vi "Calc_Force_Moment_Balance_ver2.vi"(8 "Center State at T":T2, 9 "Ini_Anchor_Posi":dbl[][](array[numeric]), 10 "Torque":dbl, 11 "On_Particle State":T1(array[cluster])) -> (0 "New Center State at T":T2, 1 "Ini_Anchor_Posi":dbl[][](array[numeric]), 2 "Rot_angle":dbl, 3 "On_Particle State":T1(array[cluster]), 4 "final Moment":dbl, 6 "initial Moment":dbl)   [LabVIEW 2020]
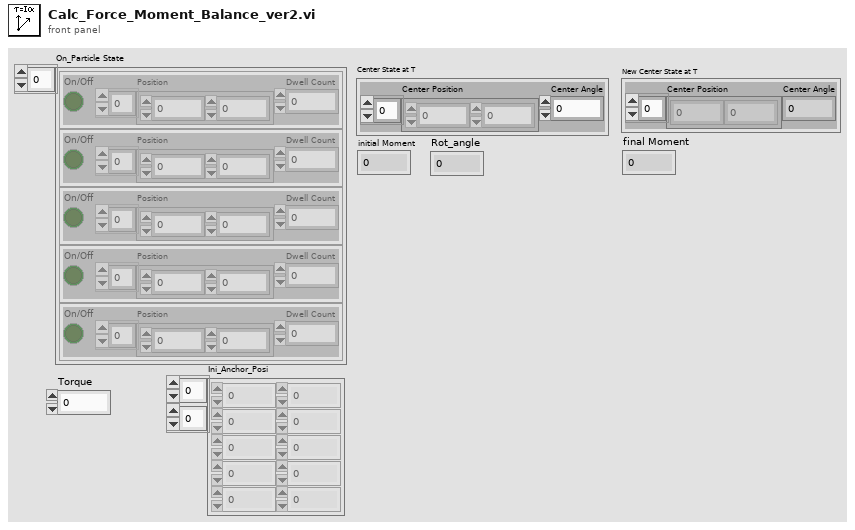
[diagram p1: front panel]
types:
  T1 = cluster{"On/Off":bool, "Position":dbl[], "Dwell Count":i32}[]
  T2 = cluster{"Center Position":dbl[], "Center Angle":dbl}
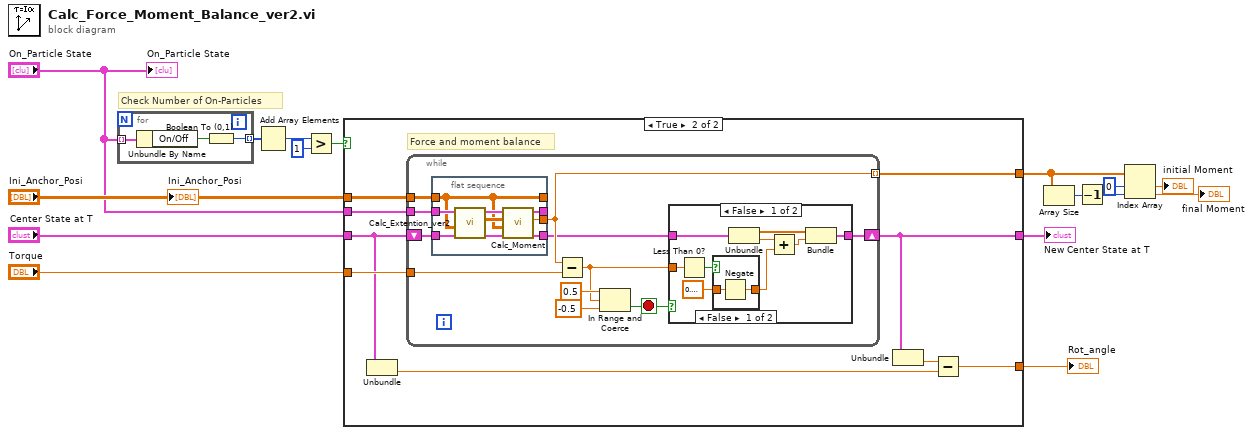
[diagram p0: block diagram]
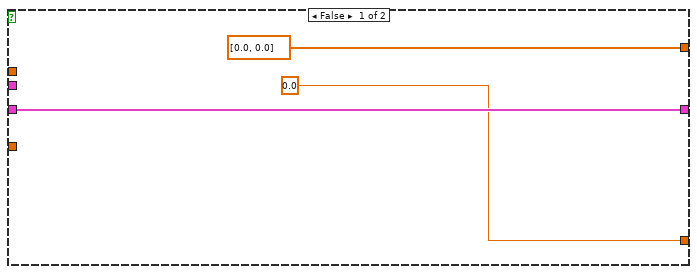
[diagram p2: hidden frame]
diagram:
  # "Check Number of On-Particles"
  n1 = for {
    tunnel: "On_Particle State" -> [w19] mode=indexing
    tunnel: [w17] -> w15 mode=indexing
    n2 = Unbundle By Name(w19) -> ("On/Off"=w18:bool)
    n3 = Boolean To (0,1)(Boolean=w18) -> (0, 1=w17:i16)
  }
  n4 = Add Array Elements(numeric array=w15) -> (sum=w9:i16)
  n5 = Greater?(x=w9, y=i16 1) -> (0:w13:bool)
  n6 = case shown="TRUE" w13 {
    tunnel: "Center State at T" -> [w22 w25]
    tunnel: "Ini_Anchor_Posi" -> [_ w30]
    tunnel: [w22 w27] -> w10
    tunnel: "On_Particle State" -> [_ w29]
    tunnel: "Torque" -> [_ w31]
    tunnel: [dbl[] [0.0, 0.0] w28] -> w4
    tunnel: [0.0 w23] -> w1
    frame False {
    }
    frame True {
      # "Force and moment balance"
      n7 = Unbundle(w25) -> ("Center Angle"=w24:dbl)  [unwired: 1 out]
      n8 = while {
        shift-right: [w35] -> w27
        shift-left: w25 -> [w42]
        tunnel: w30 -> [w41]
        tunnel: w31 -> [w39]
        tunnel: [w38] -> w28 mode=indexing
        tunnel: w29 -> [w37]
        stop <- w34 stop-if-true
        n9 = flat-sequence {
          tunnel: w41 -> [w57]
          tunnel: w42 -> [w63]
          tunnel: [w62] -> w36
          tunnel: w37 -> [w61]
          tunnel: [w60] -> w38
          tunnel: [w58] -> _
          tunnel: [w57] -> _
          frame #0 {
            n10 = call "Calc_Extention_ver2.vi"("Center State at T"=w63, "Initial Anchor Position"=w57, "On_Particle State"=w61) -> ("New Center State at T"=w56:T2, "Extension"=w59:dbl[][], "On_Particle State"=w64:T1)  [unwired: 6 in]
            n11 = call "Calc_Moment.vi"("Center State at T"=w56, "Initial Anchor Position"=w57, "Extention"=w59, "On_Particle State"=w64) -> ("Center State at T 2"=w62:T2, "SummedMoment"=w60:dbl, "On_Particle State"=w58:T1)  [unwired: 5 in]
          }
        }
        n12 = Subtract(x=w38, y=w39) -> (x-y=w33:dbl)
        n13 = In Range and Coerce(upper limit=0.5, x=w33, lower limit=-0.5) -> (In Range?=w34:bool)  [unwired: 1 out]
        n14 = case shown="FALSE" w34 {
          tunnel: w36 -> [w48 w55]
          tunnel: [w44 w55] -> w35
          tunnel: w33 -> [w43 _]
          frame False {
            n15 = Less Than 0?(x=w43) -> (x < 0?=w51:bool)
            n16 = case shown="FALSE" w51 {
              tunnel: [w52 w54] -> w49
              tunnel: 0.10000000000000003 ("y") -> [w53 w54]
              frame False {
                n17 = Negate(x=w53) -> (-x=w52:dbl)
              }
              frame True {
              }
            }
            n18 = Unbundle(w48) -> ("Center Position"=w47:dbl[], "Center Angle"=w45:dbl)
            n19 = Add(x=w45, y=w49) -> (x+y=w46:dbl)
            n20 = Bundle("Center Position"=w47, w46) -> (w44:cluster{"Center Position":dbl[], dbl})  [unwired: 1 in]
          }
          frame True {
          }
        }
      }
      n21 = Unbundle(w27) -> ("Center Angle"=w26:dbl)  [unwired: 1 out]
      n22 = Subtract(x=w26, y=w24) -> (x-y=w23:dbl)
    }
  }
  "New Center State at T" <- w10
  "Rot_angle" <- w1
  n23 = Array Size(array=w4) -> (size(s)=w6:i32)
  n24 = Decrement(x=w6) -> (x-1=w7:i32)
  n25 = Index Array(array=w4, index #1=0 ("指標"), index #2=w7) -> (element #1=→"initial Moment":dbl, element #2=→"final Moment":dbl)
  "On_Particle State" <- "On_Particle State"
  "Ini_Anchor_Posi" <- "Ini_Anchor_Posi"
